vi "Matches.vi"(8 "error in (no error)":errorcluster, 10 "Actual":variant, 11 "Collection Distinct in":refnum<class "Collection Distinct.lvclass">) -> (0 "error out":errorcluster, 2 "Result":bool, 3 "Collection Distinct out":refnum<class "Collection Distinct.lvclass">)   [LabVIEW 2017, in "Transparent Assertions.lvlib" / "Collection Distinct.lvclass"]
doc: "Evaluates the constraint for <B>Actual</B>. Returns true if the constraint is met."
uses:
  Collection Distinct.lvclass
  Transparent Assertions.lvlib
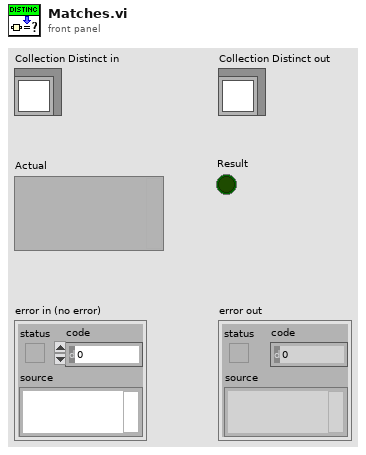
[diagram p1: front panel]
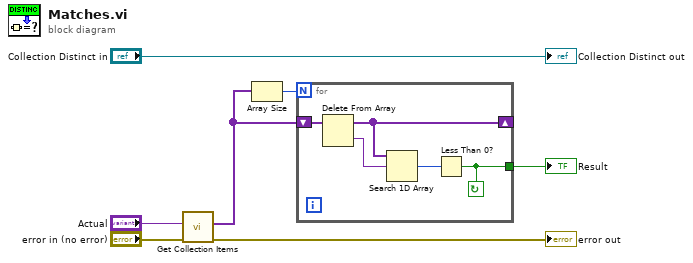
[diagram p0: block diagram]
diagram:
  n1 = call "Get Collection Items.vi"("error in (no error)"="error in (no error)", "Collection"="Actual") -> ("error out"=→"error out":errorcluster, "Items"=w1:variant[])  [unwired: 8 in]
  n2 = Array Size(array=w1) -> (size(s)=w2:i32)
  n3 = for {
    N: w2 -> [_]
    shift-right: [w9] -> _
    shift-left: w1 -> [w10]
    tunnel: [w11] -> w3
    stop <- w11 continue-if-true
    n4 = Delete From Array(array=w10) -> (deleted portion=w8:variant, array with subset deleted=w9:variant[])  [unwired: 2 in]
    n5 = Search 1D Array(1D array=w9, element=w8) -> (index of element=w12:i32)  [unwired: 1 in]
    n6 = Less Than 0?(x=w12) -> (x < 0?=w11:bool)
  }
  "Result" <- w3
  "Collection Distinct out" <- "Collection Distinct in"
